vi "Save_Picture_Log.vi"() -> (5 "Plug in titles":string[](array[string]), 7 "Plug in values":string[](array[string]))   [LabVIEW 2018]
uses:
  Controls/Post_Process.ctl
  Globals/Meas_global.vi
panel:
  out "New Log Path":path
  out "Source Path":path
  # "Run this VI to update the channel names"
  # "You Must have selected the \"Save Data\" option on the \nMeasurement Program for this vi to save the Picture log"
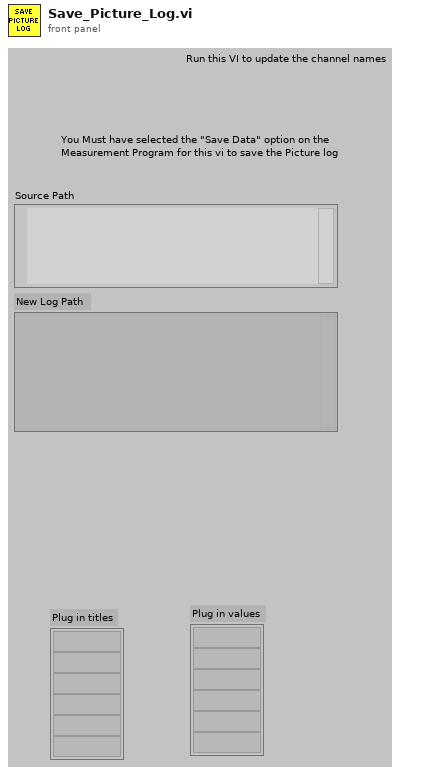
[diagram p1: front panel]
types:
  T1 = typedef "Post_Process.ctl" = enum16{"Take New Data", "Post Process Raw Data File"}
  T2 = enum16{"Save no data", "Save data in new files", "Save data in existing files"}
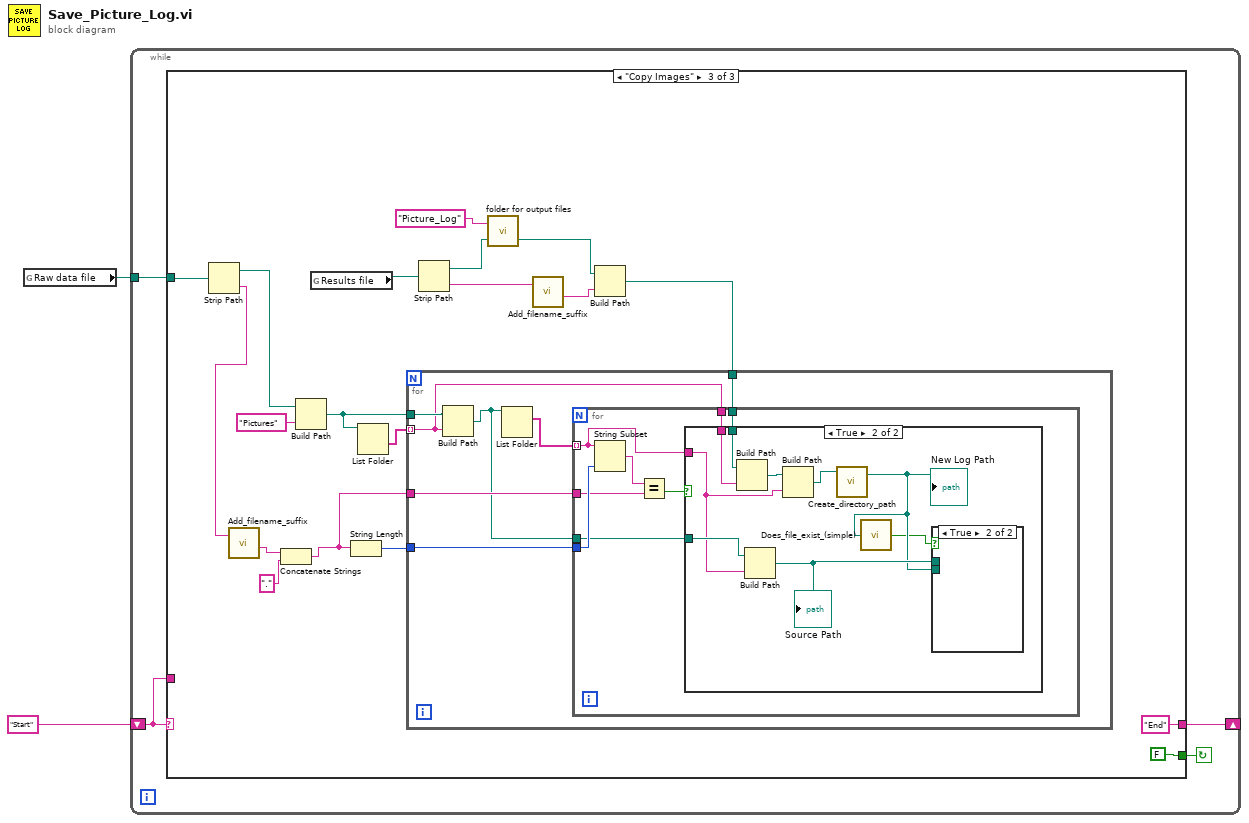
[diagram p0: block diagram]
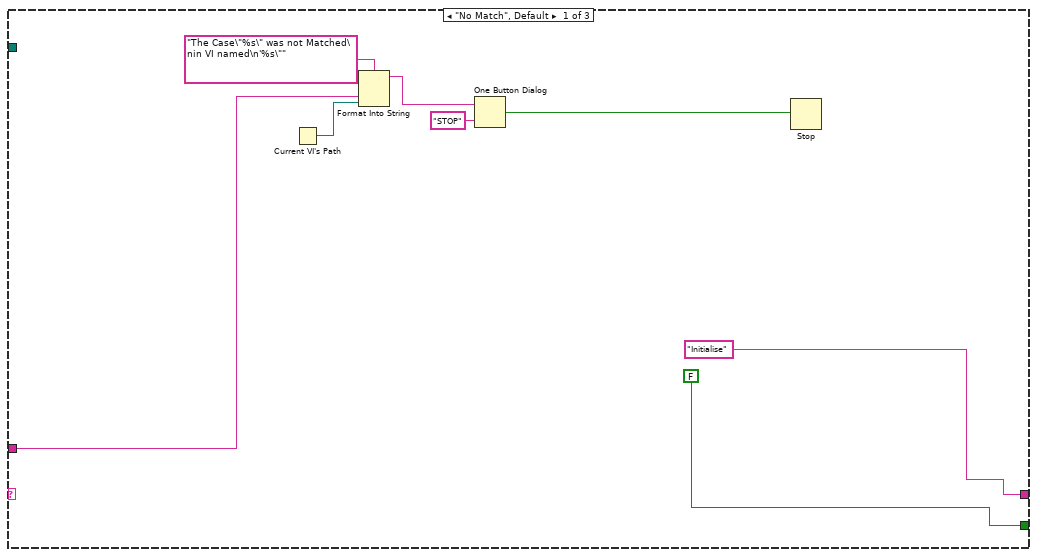
[diagram p2: hidden frame]
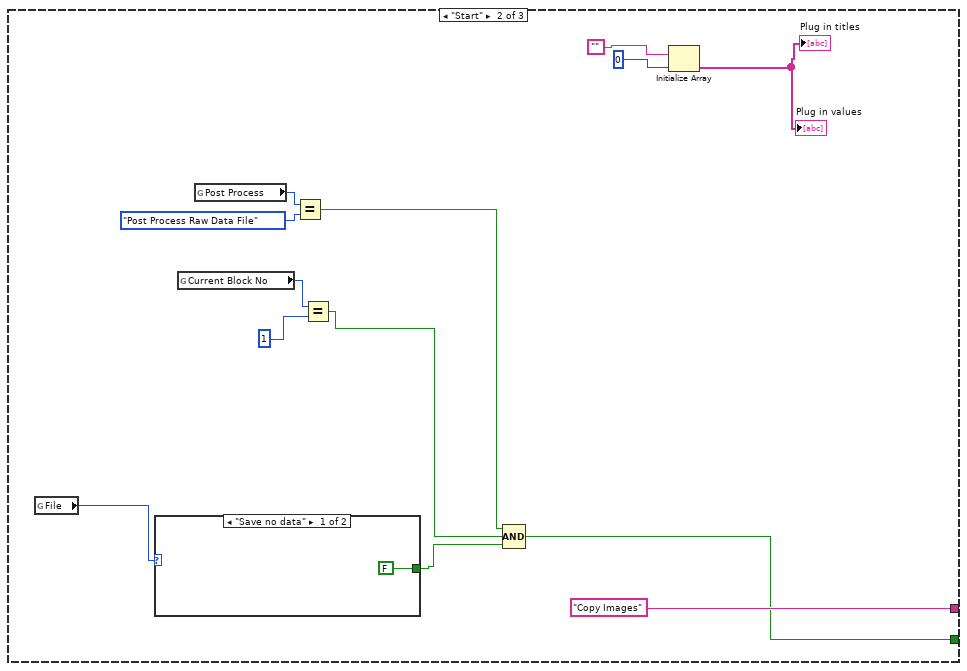
[diagram p3: hidden frame]
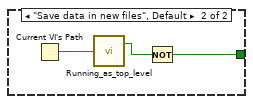
[diagram p4: hidden frame]
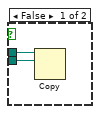
[diagram p6: hidden frame]
diagram:
  n1 = global read "Meas_global.vi" "Raw data file"() -> (w1:path)
  n2 = while {
    shift-left: "Start" -> [w4]
    shift-right: [w5] -> _
    tunnel: w1 -> [w3]
    stop <- w6 continue-if-true
    n3 = case shown="\"Copy Images\"" w4 {
      tunnel: [FALSE w19 FALSE] -> w6
      tunnel: ["Initialise" "Copy Images" ("t") "End" ("t")] -> w5
      tunnel: w4 -> [w9 _ _]
      tunnel: w3 -> [_ _ w48]
      frame "No Match", Default {
        n4 = Current VI's Path() -> (path=w8:path)
        n5 = Format Into String(format string="The Case\"%s\" was not Matched\nin VI named\n'%s\"" ("Format String"), w9, w8) -> (resulting string=w12:string)  [unwired: 2 in, 1 out]
        n6 = One Button Dialog(message=w12, button name ("OK")="STOP") -> (true=w10:bool)
        n7 = Stop(stop? (T)=w10) -> ()
      }
      frame "Start" {
        n8 = global read "Meas_global.vi" "File"() -> (w26:T2)
        n9 = case shown="\"Save no data\"" w26 {
          tunnel: [FALSE w29] -> w20
          frame "Save no data" {
          }
          frame "Save data in new files", Default {
            n10 = Current VI's Path() -> (path=w30:path)
            n11 = call "Running_as_top_level.vi"("Vi path name"=w30) -> ("Top Level"=w31:bool)  [unwired: 1 out]
            n12 = Not(x=w31) -> (.not. x?=w29:bool)
          }
        }
        n13 = global read "Meas_global.vi" "Current Block No"() -> (w23:i32)
        n14 = global read "Meas_global.vi" "Post Process"() -> (w16:T1)
        n15 = Equal?(x=w16, y=Post_Process."Post Process Raw Data File" ("Post Process")) -> (x = y?=w15:bool)
        n16 = Equal?(x=w23, y=1) -> (x = y?=w21:bool)
        n17 = Compound Arithmetic op=AND(w15, w21, w20) -> (w19:bool)
        n18 = Initialize Array("", 0) -> (→"Plug in values" →"Plug in titles":string[])
      }
      frame "Copy Images" {
        n19 = Strip Path(path=w48) -> (stripped path=w44:path, name=w40:string)
        n20 = call "Add_filename_suffix.vi"("Filename"=w40) -> ("Base name"=w37:string)  [unwired: 1 in, 3 out]
        n21 = Concatenate Strings(w37, "." ("string")) -> (w35:string)
        n22 = Build Path(base path=w44, name or relative path="Pictures") -> (appended path=w42:path)
        n23 = global read "Meas_global.vi" "Results file"() -> (w45:path)
        n24 = String Length(string=w35) -> (length=w39:i32)
        n25 = List Folder(path=w42) -> (folder names=w41:string[])  [unwired: 3 in, 3 out]
        n26 = Strip Path(path=w45) -> (stripped path=w34:path, name=w46:string)
        n27 = call "folder for output files.vi"("results folder"=w34, "folder name"="Picture_Log" ("name or relative path")) -> ("appended path"=w32:path)  [unwired: 1 out]
        n28 = call "Add_filename_suffix.vi"("Filename"=w46) -> ("Base name"=w47:string)  [unwired: 1 in, 3 out]
        n29 = Build Path(base path=w32, name or relative path=w47) -> (appended path=w38:path)
        n30 = for {
          tunnel: w42 -> [w57]
          tunnel: w41 -> [w53] mode=indexing
          tunnel: w39 -> [w55]
          tunnel: w35 -> [w54]
          tunnel: w38 -> [w52]
          n31 = Build Path(base path=w57, name or relative path=w53) -> (appended path=w51:path)
          n32 = List Folder(path=w51) -> (filenames=w56:string[])  [unwired: 3 in, 3 out]
          n33 = for {
            tunnel: w56 -> [w59] mode=indexing
            tunnel: w55 -> [w65]
            tunnel: w54 -> [w63]
            tunnel: w53 -> [w61]
            tunnel: w52 -> [w60]
            tunnel: w51 -> [w58]
            n34 = String Subset(string=w59, length (rest)=w65) -> (substring=w64:string)  [unwired: 1 in]
            n35 = Equal?(x=w64, y=w63) -> (x = y?=w62:bool)
            n36 = case shown="True" w62 {
              tunnel: w61 -> [_ w74]
              tunnel: w60 -> [_ w73]
              tunnel: w59 -> [_ w70]
              tunnel: w58 -> [_ w71]
              frame False {
              }
              frame True {
                n37 = Build Path(base path=w73, name or relative path=w74) -> (appended path=w72:path)
                n38 = Build Path(base path=w71, name or relative path=w70) -> (appended path=w68:path)
                "Source Path" <- w68
                n39 = Build Path(base path=w72, name or relative path=w70) -> (appended path=w69:path)
                n40 = call "Create_directory_path.vi"("Path name"=w69) -> ("Path name Out"=w67:path)  [unwired: 2 in, 1 out]
                "New Log Path" <- w67
                n41 = call "Does_file_exist_(simple).vi"("Pathname"=w67) -> ("exists?"=w66:bool)
                n42 = case shown="True" w66 {
                  tunnel: w68 -> [w76 _]
                  tunnel: w67 -> [w75 _]
                  frame False {
                    n43 = Copy(10:w75, 11:w76) -> ()  [unwired: 3 in, 3 out]
                  }
                  frame True {
                  }
                }
              }
            }
          }
        }
      }
    }
  }
